vi "Setup.vi"(11 "Network Sink Endpoint in":refnum<class "Network Sink Endpoint.lvclass">) -> (0 "error out":errorcluster, 3 "Network Sink Endpoint out":refnum<class "Network Sink Endpoint.lvclass">)   [LabVIEW 2017, in "Network Sink.lvlib" / "Network Sink Endpoint.lvclass"]
uses:
  <vilib>/gpm_packages/@cs/event-logger/Source/Network Sink/Network Sink Endpoint/Network Sink Endpoint.lvclass
  <vilib>/gpm_packages/@cs/event-logger/Source/Network Sink/LogEventMessageProtocol/LogEventMessageProtocol.lvclass
  C:/Program Files/National Instruments/LabVIEW 2017/vi.lib/gpm_packages/@cs/Network-Sink/Source/Network Interface/IMessagingProtocol/IMessagingProtocol.lvclass
  <vilib>/gpm_packages/@cs/event-logger/Source/Network Sink/Network Sink Endpoint/Network Sink Endpoint.lvclass/Network Sink Endpoint.ctl
  <vilib>/gpm_packages/@cs/event-logger/Source/Composed Log/LoggerReference/LoggerReference.lvclass/LoggerReference.ctl
  f6aa21b2-fdcf-4a7f-83f3-13aaa020a876.vi
  <vilib>/gpm_packages/@cs/event-logger/Source/Composed Log/LoggerReference/Send Add Sink.vi
  <vilib>/gpm_packages/@cs/event-logger/Source/Network Sink/Shutdown Sink/Shutdown Sink.lvclass
  C:/Program Files/National Instruments/LabVIEW 2017/vi.lib/gpm_packages/@cs/event-logger/Source/Composed Log/Log Sink/Log Sink.lvclass
  <vilib>/gpm_packages/@cs/Network-Sink/Source/TCP Interface/TCP Server/TCP Server.lvclass
  C:/Program Files/National Instruments/LabVIEW 2017/vi.lib/gpm_packages/@cs/Network-Sink/Source/Network Interface/IConnectionFactory/IConnectionFactory.lvclass
  <vilib>/gpm_packages/@cs/event-logger/Source/Composed Log/Log Sink/Log Sink.lvclass
  <vilib>/gpm_packages/@cs/Network-Sink/Source/Network Interface/Network Interface/Network Interface.lvclass
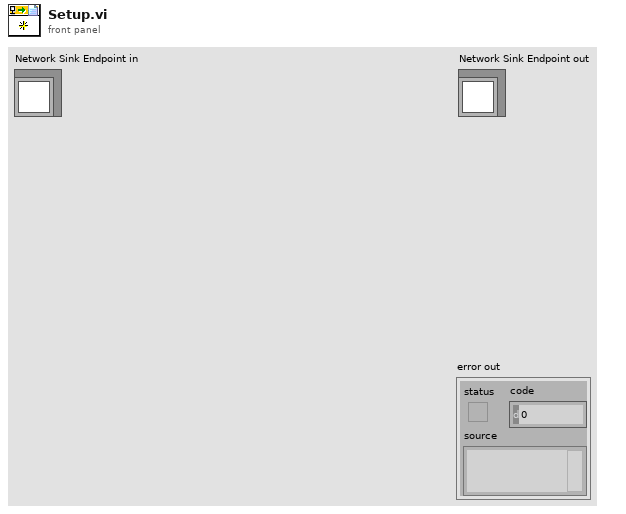
[diagram p1: front panel]
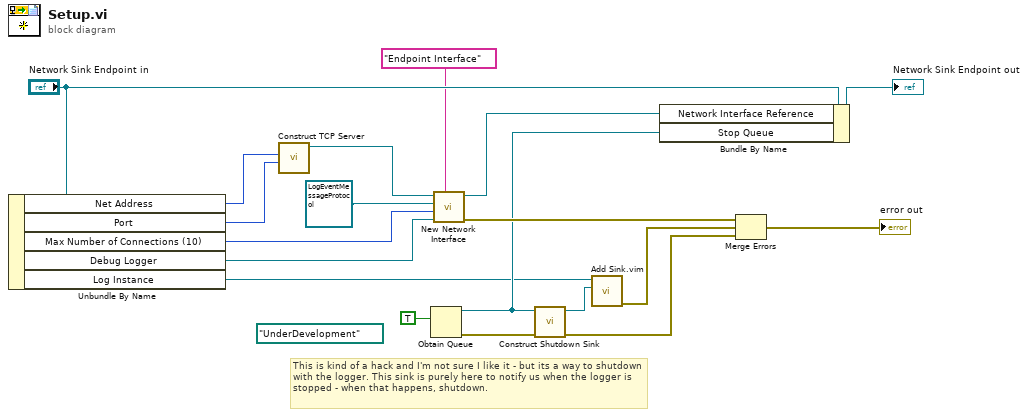
[diagram p0: block diagram]
diagram:
  (unwired) path "UnderDevelopment"
  # "This is kind of a hack and I'm not sure I like it - but its a way to shutdown with the logger. This sink is purely here to notify us when the logger is stopped - when that happens, shutdown."
  n1 = Unbundle By Name("Network Sink Endpoint in") -> ("Net Address"=w16:u32, "Port"=w15:u16, "Max Number of Connections (10)"=w14:i32, "Debug Logger"=w3:refnum<class "LoggerReference.lvclass">, "Log Instance"=w2:refnum<class "LoggerReference.lvclass">)
  n2 = call <vilib>:"Construct TCP Server.vi"("Port"=w15, "Net Address"=w16) -> ("TCP Server out"=w18:refnum<class "TCP Server.lvclass">)  [unwired: 9 in]
  n3 = Obtain Queue(element data type=TRUE) -> (queue out=w7:refnum<queue>, error out=w5:errorcluster)  [unwired: 4 in, 1 out]
  n4 = call <vilib>:"New Network Interface.vi"("Log Alias"="Endpoint Interface", "Log Instance"=w3, "Max Number of Connections to Create (1)"=w14, "MessageProtocol"=refnum<class "LogEventMessageProtocol.lvclass"> refnum ("Network Sink.lvlib:LogEventMessageProtocol.lvclass"), "Connection Factory Type"=w18) -> ("error out"=w9:errorcluster, "Network Interface Reference"=w11:refnum<data-value>)  [unwired: 5 in]
  n5 = call <vilib>:"Construct Shutdown Sink.vi"("Stop Queue"=w7) -> ("Shutdown Sink out"=w1:refnum<class "Shutdown Sink.lvclass">)  [unwired: 10 in]
  n6 = call "Add Sink.vim"("Log Sink(s)"=w1, "Log Instance In"=w2) -> ("error out"=w6:errorcluster)  [unwired: 7 in, 2 out]
  n7 = Bundle By Name(cluster="Network Sink Endpoint in", "Network Interface Reference"=w11, "Stop Queue"=w7) -> (→"Network Sink Endpoint out":refnum<class "Network Sink Endpoint.lvclass">)
  n8 = Merge Errors(w9, w6, w5) -> (→"error out":errorcluster)
